vi "Fetch Measurement Data.vi"(6 "Data Format (0 : Binary)":i32(ring) items=["Binary", "ASCII"], 8 "error in (no error)":errorcluster, 9 "End Channel (1)":string="0001", 10 "Start Channel (1)":string="0001", 11 "VISA resource name":refnum<visa-resource-name>) -> (0 "error out":errorcluster, 2 "Measurement Data":string, 3 "VISA resource name out":refnum<visa-resource-name>)   [LabVIEW 2020, in "Yokogawa GX Series.lvlib"]
doc: "Reads the measurement Binary or ASCII data of specified start to end channel numbers."
uses:
  <instrlib>/Yokogawa GX Series/Yokogawa GX Series.lvlib
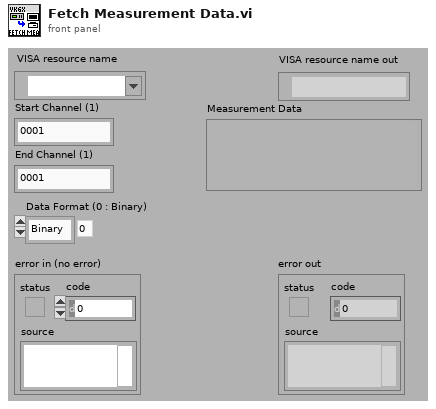
[diagram p1: front panel]
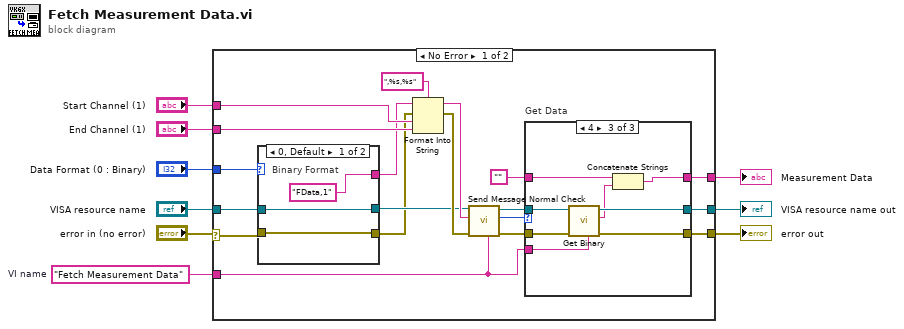
[diagram p0: block diagram]
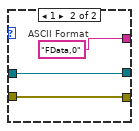
[diagram p2: hidden frame]
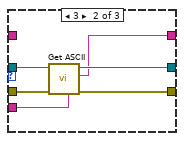
[diagram p4: hidden frame]
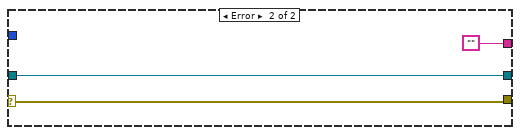
[diagram p5: hidden frame]
diagram:
  w5 = "Fetch Measurement Data"  # VI name
  n1 = case shown="No Error" "error in (no error)" {
    selector: "error in (no error)" -> [w10 w53]
    tunnel: [w28 w54] -> w9
    tunnel: [w27 w53] -> w8
    tunnel: [w26 ""] -> w7
    tunnel: "VISA resource name" -> [w23 w54]
    tunnel: w5 -> [w20 _]
    tunnel: "Start Channel (1)" -> [w19 _]
    tunnel: "End Channel (1)" -> [w18 _]
    tunnel: "Data Format (0 : Binary)" -> [w11 _]
    frame No Error {
      n2 = case shown="0, Default" w11 {
        tunnel: w23 -> [w30 w32]
        tunnel: w10 -> [w29 w33]
        tunnel: [w30 w32] -> w17
        tunnel: [w29 w33] -> w16
        tunnel: ["FData,1" "FData,0"] -> w12
        frame 0, Default {
          # "Binary Format"
        }
        frame 1 {
          # "ASCII Format"
        }
      }
      n3 = Format Into String(format string=",%s,%s", initial string=w12, error in=w16, w19, w18) -> (resulting string=w22:string, error out=w21:errorcluster)
      n4 = call <instrlib>:"Send Message Normal Check.vi"("Source (\"\")"=w20, "error in (no error)"=w21, "Send Message (\"\")"=w22, "VISA resource name"=w17) -> ("error out"=w14:errorcluster, "Response Type"=w13:i32, "VISA resource name out"=w15:refnum<visa-resource-name>)  [unwired: 1 in, 4 out]
      n5 = case "Get Data" shown="4" w13 {
        tunnel: [w37 w38 w48] -> w26
        tunnel: [w35 w40 w46] -> w27
        tunnel: [w36 w41 w51] -> w28
        tunnel: w15 -> [w36 w43 w50]
        tunnel: w14 -> [w35 w42 w47]
        tunnel: "" -> [w37 _ w49]
        tunnel: w20 -> [_ w39 w45]
        frame 0, Default {
        }
        frame 3 {
          n6 = call <instrlib>:"Get ASCII.vi"("Source (\"\")"=w39, "error in (no error)"=w42, "VISA resource name"=w43) -> ("error out"=w40:errorcluster, "ASCII Data"=w38:string, "VISA resource name out"=w41:refnum<visa-resource-name>)  [unwired: 6 out]
        }
        frame 4 {
          n7 = call <instrlib>:"Get Binary.vi"("Source (\"\")"=w45, "error in (no error)"=w47, "VISA resource name"=w50) -> ("error out"=w46:errorcluster, "Binary Data"=w44:string, "VISA resource name out"=w51:refnum<visa-resource-name>)  [unwired: 6 out]
          n8 = Concatenate Strings(w49, w44) -> (w48:string)
        }
      }
    }
    frame Error {
    }
  }
  "error out" <- w8
  "VISA resource name out" <- w9
  "Measurement Data" <- w7
